vi "newTestStandPassFailStep.vi"(0 "Engine Reference":refnum<k7>, 3 "Precondition":string, 5 "Sequence File Ref":refnum<k7>, 7 "Step Name":string="num limit test", 9 "Requirement":string, 11 "error in":errorcluster, 12 "index":i32) -> (4 "Engine reference(out)":refnum<k7>, 6 "Sequence File Ref(out)":refnum<k7>, 15 "error out":errorcluster)   [LabVIEW 2010]
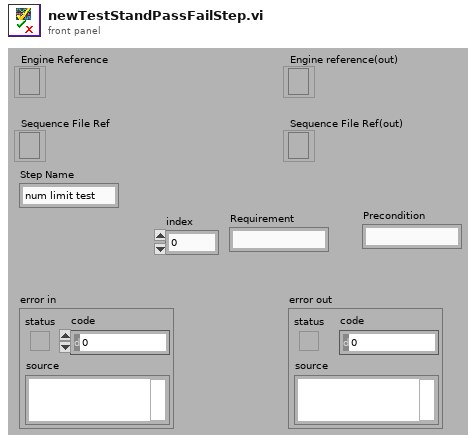
[diagram p1: front panel]
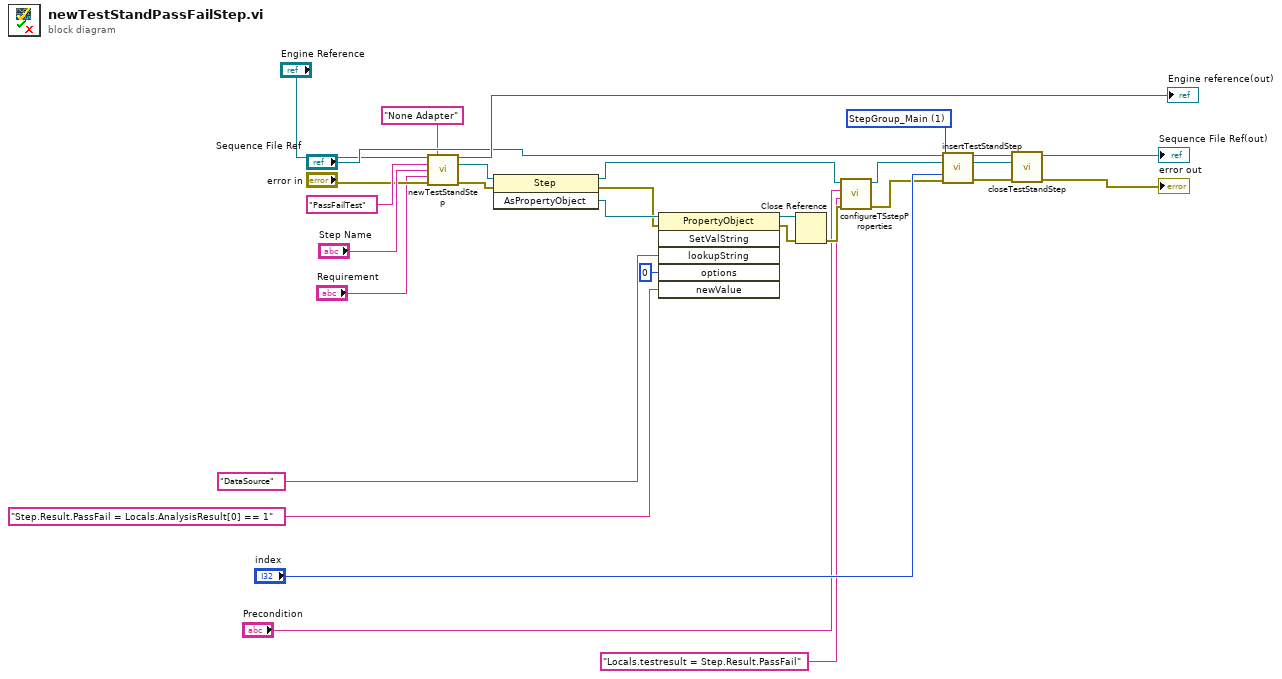
[diagram p0: block diagram]
diagram:
  w22 = 1 items=["StepGroup_Setup", "StepGroup_Main", "StepGroup_Cleanup"] ("Step Group")
  n1 = call "newTestStandStep.vi"("Engine reference"="Engine Reference", "adapterKeyNameVal"="None Adapter", "stepType"="PassFailTest", "Step Name"="Step Name", "Requirement"="Requirement", "error in"="error in") -> ("Engine reference(out)"=→"Engine reference(out)":refnum<k7>, "NewStep (out)"=w29:refnum<k7>, "error out"=w30:errorcluster)  [unwired: 7 in]
  n2 = invoke class="Step" method="AsPropertyObject"(reference=w29, error in=w30) -> (reference out=w6:refnum<k7>, error out=w1:errorcluster, "AsPropertyObject"=w2:refnum<k7>)  [unwired: 1 in]
  n3 = invoke class="PropertyObject" method="SetValString"(reference=w2, error in=w1, "lookupString"="DataSource", "options"=0, "newValue"="Step.Result.PassFail = Locals.AnalysisResult[0] == 1") -> (reference out=w13:refnum<k7>, error out=w12:errorcluster)  [unwired: 1 in, 4 out]
  n4 = Close Reference(reference=w13, error in (no error)=w12) -> (error out=w8:errorcluster)
  n5 = call "configureTSstepProperties.vi"("error in"=w8, "PostExpression"="Locals.testresult = Step.Result.PassFail", "Precondition"="Precondition", "NewStep (in)"=w6) -> ("error out"=w7:errorcluster, "NewStep (out)"=w5:refnum<k7>)  [unwired: 6 in]
  n6 = call "insertTestStandStep.vi"("Sequence File Ref"="Sequence File Ref", "Step to insert"=w5, "Step Group"=w22, "index"="index", "error out"=w7) -> ("Sequence File Ref(out)"=w25:refnum<k7>, "Step to insert (out)"=w24:refnum<k7>, "error out"=w23:errorcluster)  [unwired: 8 in]
  n7 = call "closeTestStandStep.vi"("error in"=w23, "NewStep"=w24, "Sequence File Ref"=w25) -> ("error out"=→"error out":errorcluster, "Sequence File Ref(out)"=→"Sequence File Ref(out)":refnum<k7>)  [unwired: 7 in]
